vi "TDS 2004B Three Channel Initialize SubVI w- Avg 01.vi"(0 "VISA Refnum in":refnum<visa-resource-name>, 1 "Probe Attenuation Ch A":dbl, 2 "Probe Attenuation Ch B":dbl, 3 "Trigger Source":u16, 4 "Channel B":u16, 5 "Vertical Range Ch B (V/Div)":dbl, 6 "Vertical Offset Ch B (V)":dbl, 7 "error in":errorcluster, 8 "Vertical Coupling":u16, 9 "Trigger Level (-4.4 V) in":dbl, 10 "Vertical Range Ch A (V/Div)":dbl, 11 "Trigger Mode":u16, 12 "Vertical Offset Ch A (V)":dbl, 13 "Trigger Slope":i32, 14 "Channel A":u16, 15 "Timebase":dbl=0.01 format="%#_13g", 16 "Serial Configuration 3":T1, 17 "Number of Averaged Waveforms (4: 4)":i32(ring)=128 items=["4"=4, "16"=16, "64"=64, "128"=128], 19 "Acquisition Type (0: Sample)":i32(ring)=1 items=["Sample", "Average", "Peak Detect"], 22 "Channel C":i32(ring) items=["Channel 1", "Channel 2", "Channel 3", "Channel 4", "Math", "Reference A", "Reference B", "Reference C", "Reference D"], 23 "Probe Attenuation Ch C":i32(ring)=10 items=["1"=1, "10"=10, "20"=20, "50"=50, "100"=100, "500"=500, "1000"=1000], 25 "Vertical Range Ch C (V/Div)":dbl=10.0, 26 "Vertical Offset Ch C (V)":dbl) -> (18 "Array":u16[](array[numeric]), 20 "VISA Refnum out":refnum<visa-resource-name>, 21 "Timeout (ms)":u32, 27 "error out":errorcluster)   [LabVIEW 2017]
uses:
  <instrlib>/Tektronix TDS 200 1000 2000 Series/Public/Configure/Configure Trigger (Edge).vi
  <instrlib>/Tektronix TDS 200 1000 2000 Series/Tektronix TDS 200 1000 2000 Series.lvlib
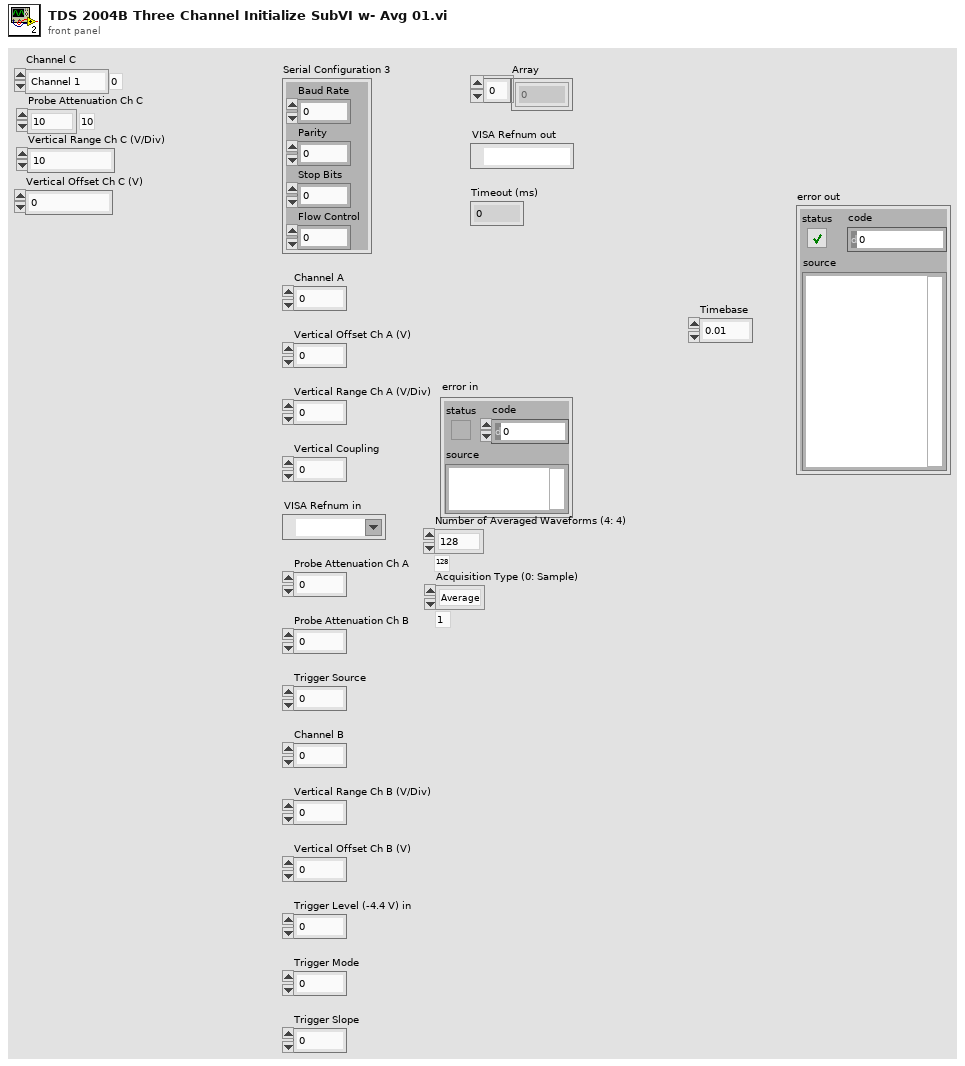
[diagram p1: front panel]
types:
  T1 = cluster{"Baud Rate":u32, "Parity":u16, "Stop Bits":u16, "Flow Control":u16}
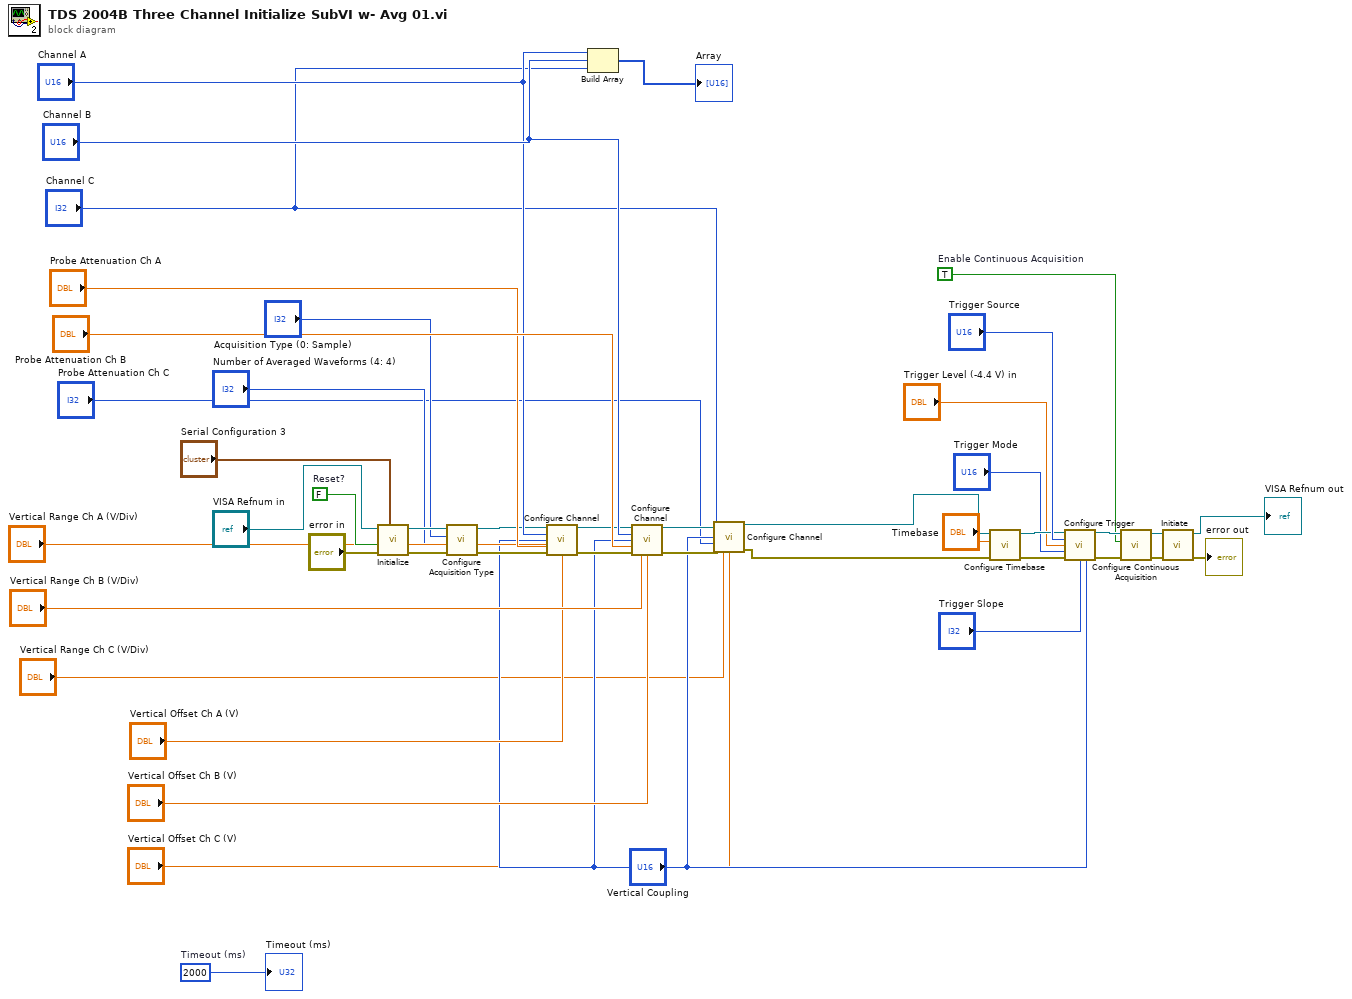
[diagram p0: block diagram]
diagram:
  w23 = FALSE  # Reset?
  w32 = u32 2000  # Timeout (ms)
  w19 = TRUE  # Enable Continuous Acquisition
  n1 = call <instrlib>:"Initialize.vi"("Serial Configuration"="Serial Configuration 3", "error in (no error)"="error in", "Reset? (T: Yes)"=w23, "VISA resource name"="VISA Refnum in") -> ("error out"=w15:errorcluster, "VISA resource name out"=w13:refnum<visa-resource-name>)  [unwired: 6 in]
  n2 = call <instrlib>:"Configure Acquisition Type.vi"("error in (no error)"=w15, "Number of Averaged Waveforms (4: 4)"="Number of Averaged Waveforms (4: 4)", "Acquisition Type (0: Sample)"="Acquisition Type (0: Sample)", "VISA resource name"=w13) -> ("error out"=w14:errorcluster, "VISA resource name out"=w12:refnum<visa-resource-name>)  [unwired: 6 in]
  n3 = call <instrlib>:"Configure Channel.vi"("VISA resource name"=w12, "Channel (0: Channel 1)"="Channel A", "Vertical Coupling (1: DC)"="Vertical Coupling", "Probe Attenuation (10: 10X)"="Probe Attenuation Ch A", "error in (no error)"=w14, "Vertical Range (10.0 V/div)"="Vertical Range Ch A (V/Div)", "Vertical Offset (0.0 divs)"="Vertical Offset Ch A (V)") -> ("VISA resource name out"=w37:refnum<visa-resource-name>, "error out"=w40:errorcluster)  [unwired: 7 in]
  n4 = Build Array("Channel A", "Channel B", "Channel C") -> (→"Array":i32[])
  n5 = call <instrlib>:"Configure Channel.vi"("VISA resource name"=w37, "Channel (0: Channel 1)"="Channel B", "Vertical Coupling (1: DC)"="Vertical Coupling", "Probe Attenuation (10: 10X)"="Probe Attenuation Ch B", "error in (no error)"=w40, "Vertical Range (10.0 V/div)"="Vertical Range Ch B (V/Div)", "Vertical Offset (0.0 divs)"="Vertical Offset Ch B (V)") -> ("VISA resource name out"=w9:refnum<visa-resource-name>, "error out"=w8:errorcluster)  [unwired: 7 in]
  n6 = call <instrlib>:"Configure Channel.vi"("VISA resource name"=w9, "Channel (0: Channel 1)"="Channel C", "Vertical Coupling (1: DC)"="Vertical Coupling", "Probe Attenuation (10: 10X)"="Probe Attenuation Ch C", "error in (no error)"=w8, "Vertical Range (10.0 V/div)"="Vertical Range Ch C (V/Div)", "Vertical Offset (0.0 divs)"="Vertical Offset Ch C (V)") -> ("VISA resource name out"=w7:refnum<visa-resource-name>, "error out"=w6:errorcluster)  [unwired: 7 in]
  n7 = call <instrlib>:"Configure Timebase.vi"("error in (no error)"=w6, "Timebase (0.0005 s)"="Timebase", "VISA resource name"=w7) -> ("error out"=w26:errorcluster, "VISA resource name out"=w25:refnum<visa-resource-name>)  [unwired: 7 in]
  n8 = call-poly <instrlib>:"Configure Trigger.vi"("VISA resource name"=w25, "Trigger Source (0: Channel 1)"="Trigger Source", "Trigger Level (0.0 V)"="Trigger Level (-4.4 V) in", "Trigger Mode (0: Auto)"="Trigger Mode", "error in (no error)"=w26, "Trigger Slope (0: Rising)"="Trigger Slope", "Trigger Coupling (0: AC)"="Vertical Coupling") -> ("VISA resource name out"=w27:refnum<visa-resource-name>, "error out"=w28:errorcluster)  [unwired: 7 in]
  n9 = call <instrlib>:"Configure Continuous Acquisition.vi"("error in (no error)"=w28, "Enable Continuous Acquisition Mode (True)"=w19, "VISA resource name"=w27) -> ("error out"=w31:errorcluster, "VISA resource name out"=w29:refnum<visa-resource-name>)  [unwired: 7 in]
  n10 = call <instrlib>:"Initiate.vi"("error in (no error)"=w31, "VISA resource name"=w29) -> ("error out"=→"error out":errorcluster, "VISA resource name out"=→"VISA Refnum out":refnum<visa-resource-name>)  [unwired: 8 out]
  "Timeout (ms)" <- w32
